vi "Swerve Controller Initialization.vi"(10 "Subsystem Name":string, 11 "Default Command":T1 {"CHASSIS"."vOmega" format="%10.3f"; "CHASSIS"."vY" format="%10.3f"; "CHASSIS"."vX" format="%10.3f"}) -> (3 "Current Command":T7 {"Current Command"."CHASSIS"."vOmega" format="%10.3f"; "Current Command"."CHASSIS"."vY" format="%10.3f"; "Current Command"."CHASSIS"."vX" format="%10.3f"; "Command Arguments"."Default Command"."CHASSIS"."vOmega" format="%10.3f"; "Command Arguments"."Default Command"."CHASSIS"."vY" format="%10.3f"; "Command Arguments"."Default Command"."CHASSIS"."vX" format="%10.3f"})   [LabVIEW 2023]
doc: "This VI is called once for the subsystem. It allocates the notifier and combines the timing, default command, and other information into a single data wire."
uses:
  Swerve Setpoints.ctl
  Swerve Operations.ctl
  <vilib>/Rock Robotics/WPI/ThirdParty/JAS_Junk/TrajLib/TypeDef/CHASSIS_SPEEDS.ctl
  <vilib>/Rock Robotics/WPI/Framework/Command Status Info.ctl
  <vilib>/Rock Robotics/WPI/Framework/Completion Status.ctl
  <vilib>/Rock Robotics/WPI/Framework/Completion Notifier.ctl
  Swerve Published Globals.vi
  <vilib>/Rock Robotics/WPI/ThirdParty/JAS_Junk/TrajLib/Trajectory_Library.lvlib
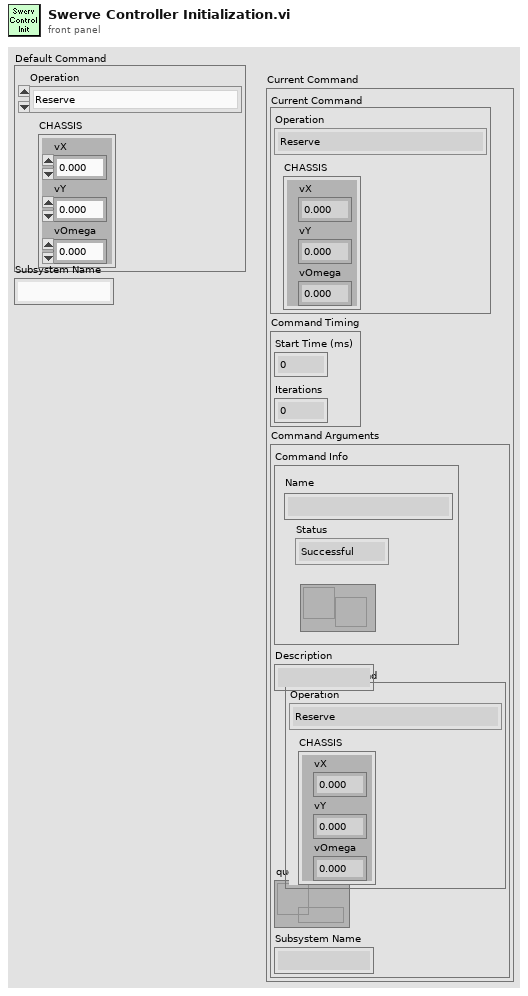
[diagram p1: front panel]
types:
  T1 = typedef "Swerve Setpoints.ctl" = cluster{"Operation":T2, "CHASSIS":T3}
  T2 = typedef "Swerve Operations.ctl" = enum16{"Reserve", "Read Current", "Immediate", "Joystick Drive"}
  T3 = typedef "Trajectory_Library.lvlib/CHASSIS_SPEEDS.ctl" = cluster{"vX":dbl, "vY":dbl, "vOmega":dbl}
  T4 = typedef "Command Status Info.ctl" = cluster{"Name":string, "Status":T5, "notifier out":T6}
  T5 = typedef "Completion Status.ctl" = enum16{"Successful", "Aborted", "Incomplete"}
  T6 = typedef "Completion Notifier.ctl" = refnum<notifier>
  T7 = cluster{"Current Command":T1, "Command Timing":cluster{"Start Time (ms)":u32, "Iterations":i32}, "Command Arguments":cluster{"Command Info":T4, "Description":string, "Default Command":T1, "queue out":refnum<queue>, "Subsystem Name":string}}
  T8 = cluster{"Default Command":T1, "Command Info":T4, "Description":string}
  T9 = cluster{"Command Info":T4, "Description":string, "Default Command":T1, "queue out":refnum<queue>, "Subsystem Name":string}
  T10 = cluster{"Default Command":T1, cluster{"Start Time (ms)":u32, "Iterations":i32}, cluster{"Command Info":T4, "Description":string, "Default Command":T1, "queue out":refnum<queue>, "Subsystem Name":string}}
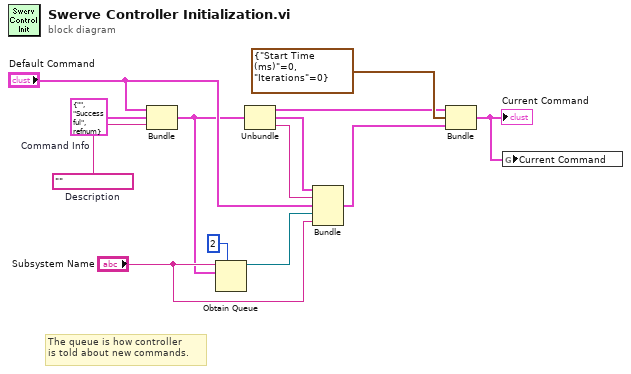
[diagram p0: block diagram]
diagram:
  w10 = T4 {"Name"="", "Status"=enum."Successful", "notifier out"=refnum}  # Command Info
  w11 = ""  # Description
  # "The queue is how controller\nis told about new commands."
  n1 = Bundle("Default Command"="Default Command", "Command Info"=w10, "Description"=w11) -> (w4:T8)  [unwired: 1 in]
  n2 = Obtain Queue(max queue size (-1, unlimited)=2, name (unnamed)="Subsystem Name", element data type=w4) -> (queue out=w3:refnum<queue>)  [unwired: 2 in, 2 out]
  n3 = Unbundle(w4) -> ("Default Command"=w12:T1, "Command Info"=w7:T4, "Description"=w8:string)
  n4 = Bundle("Command Info"=w7, "Description"=w8, "Default Command"="Default Command", "queue out"=w3, "Subsystem Name"="Subsystem Name") -> (w9:T9)  [unwired: 1 in]
  n5 = Bundle("Default Command"=w12, cluster{"Start Time (ms)":u32, "Iterations":i32} {"Start Time (ms)"=0, "Iterations"=0}, w9) -> (w1:T10)  [unwired: 1 in]
  "Current Command" <- w1
  n6 = global write "Swerve Published Globals.vi" "Current Command"(w1) -> ()
